vi "BWC_analogSamplePFFT.vi"() -> ()   [LabVIEW 2017]
uses:
  <vilib>/VirtualBench/_MSO Configure Analog Channel0.vi
  <vilib>/VirtualBench/_MSO Configure Timing8.vi
  <vilib>/measure/maspectr.llb/FFT Power Spectrum and PSD for N Chan.vi
  <vilib>/VirtualBench/VirtualBench.lvlib
  <vilib>/measure/NI_MAPro.lvlib
panel:
  in  "stop":bool
  in  "averaging parameters":T1={"averaging mode"=enum."No averaging", "weighting mode"=enum."Exponential", "number of averages"=10} {"number of averages" min=1}
  out "Power Spectrum / PSD":cluster{"f0":dbl, "df":dbl, "magnitude":dbl[]}[](graph)
  out "size(s)":i32
  in  "Auto Trigger":bool caption="Auto Trigger (False)"
  in  "Pretrigger Time (s)":dbl=0.5 caption="Pretrigger Time (s) (no change)"
  in  "Acquisition Time (s)":dbl=1.0 caption="Acquisition Time (s) (no change)"
  in  "Sample Rate":dbl=100000.0 caption="Sample Rate (no change)"
  in  "Vertical Range":dbl=1.0 caption="Vertical Range (no change)"
  in  "Vertical Offset":dbl caption="Vertical Offset (no change)"
  in  "Probe Attenuation":i32(ring)=1 caption="Probe Attenuation (no change)" items=["1x"=1, "10x"=10]
  in  "Vertical Coupling":i32(ring)=1 caption="Vertical Coupling (no change)" items=["AC", "DC"]
  in  "Enable Channel":bool=TRUE caption="Enable Channel (no change)"
  in  "Channel":tag
  out "Analog Waveforms":dynamicdata(graph)
  out "Error Out":errorcluster
  in  "Device Name":tag
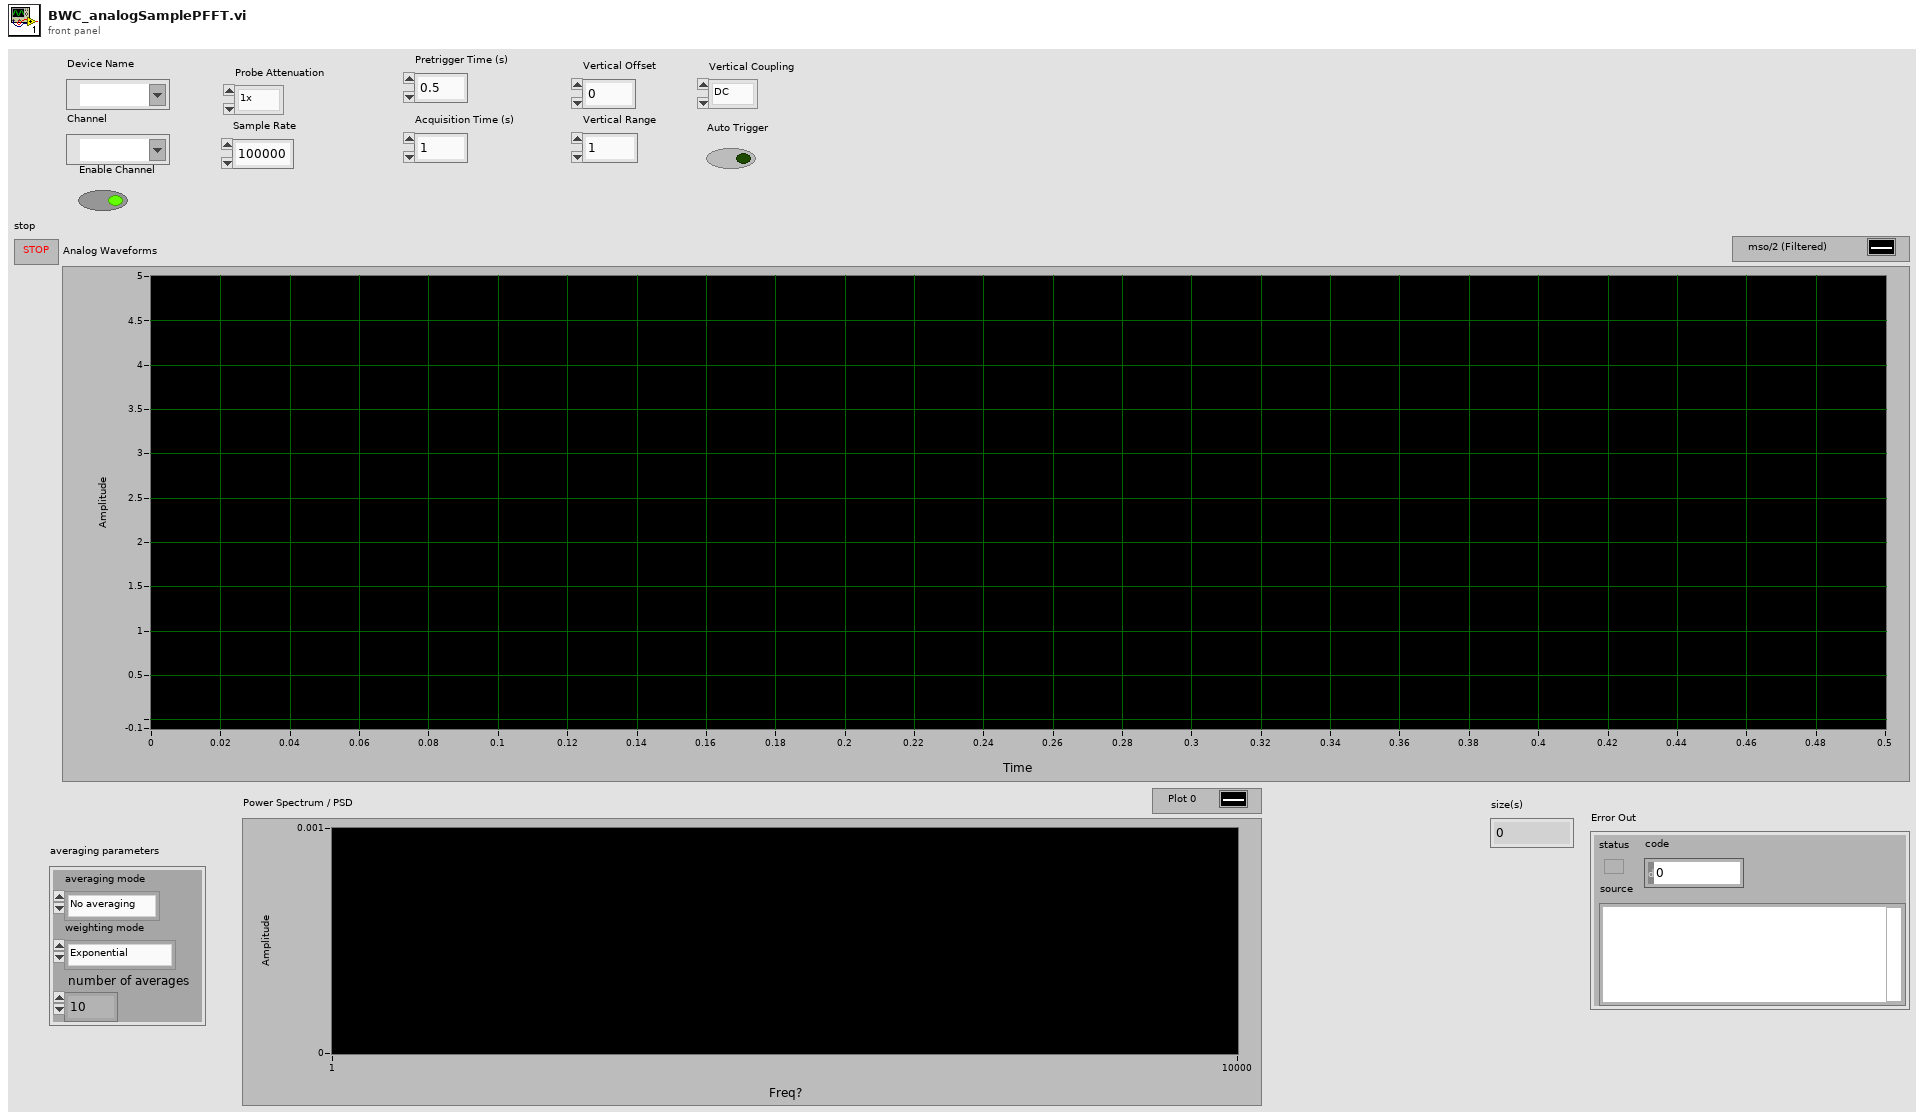
[diagram p1: front panel]
types:
  T1 = cluster{"averaging mode":enum16{"No averaging", "Vector averaging", "RMS averaging", "Peak hold"}, "weighting mode":enum16{"Linear", "Exponential"}, "number of averages":u32}
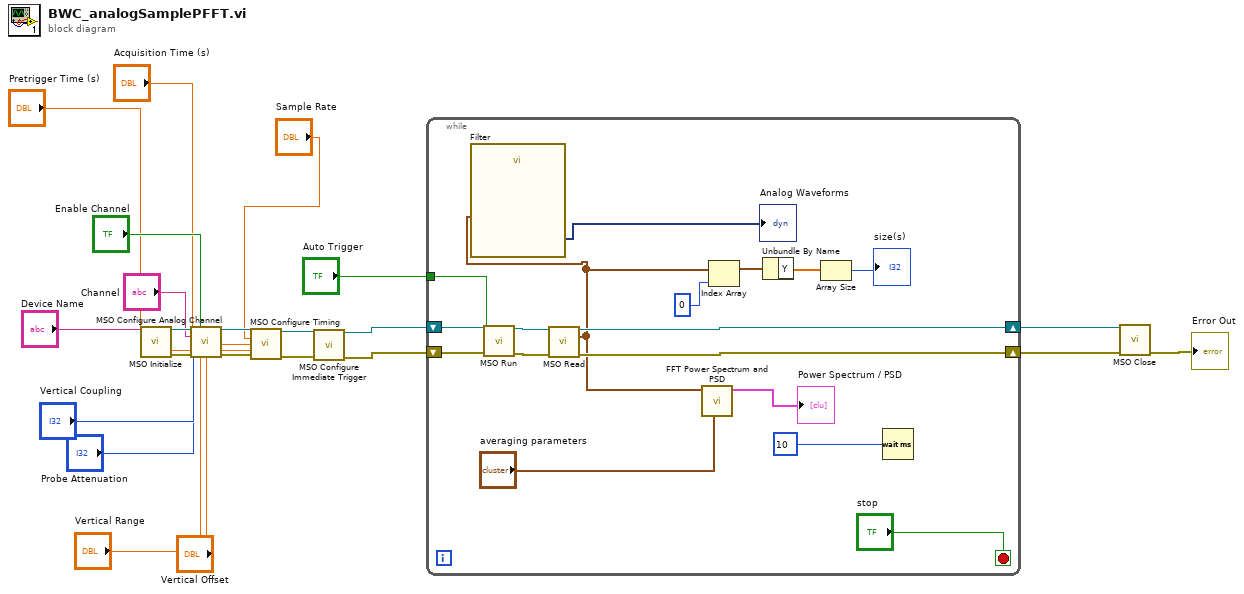
[diagram p0: block diagram]
diagram:
  n1 = call <vilib>:"MSO Initialize.vi"("Device Name"="Device Name") -> ("Instrument Handle Out"=w18:refnum<k21>, "Error Out"=w17:errorcluster)  [unwired: 13 in]
  n2 = call-poly <vilib>:"MSO Configure Analog Channel.vi"("Instrument Handle In"=w18, "Enable Channel"="Enable Channel", "Channel"="Channel", "Vertical Coupling"="Vertical Coupling", "Probe Attenuation"="Probe Attenuation", "Error In"=w17, "Vertical Range"="Vertical Range", "Vertical Offset"="Vertical Offset") -> ("Instrument Handle Out"=w15:refnum<k21>, "Error Out"=w12:errorcluster)  [unwired: 6 in]
  n3 = call-poly <vilib>:"MSO Configure Timing.vi"("Instrument Handle In"=w15, "Sample Rate"="Sample Rate", "Acquisition Time (s)"="Acquisition Time (s)", "Pretrigger Time (s)"="Pretrigger Time (s)", "Error In"=w12) -> ("Instrument Handle Out"=w14:refnum<k21>, "Error Out"=w11:errorcluster)  [unwired: 9 in]
  n4 = call <vilib>:"MSO Configure Immediate Trigger.vi"("Instrument Handle In"=w14, "Error In"=w11) -> ("Instrument Handle Out"=w13:refnum<k21>, "Error Out"=w10:errorcluster)  [unwired: 12 in]
  n5 = while {
    tunnel: "Auto Trigger" -> [w33]
    shift-right: [w39] -> w21
    shift-left: w13 -> [w37]
    shift-right: [w38] -> w20
    shift-left: w10 -> [w35]
    stop <- "stop" stop-if-true
    n6 = call <vilib>:"MSO Run.vi"("Instrument Handle In"=w37, "Auto Trigger"=w33, "Error In"=w35) -> ("Instrument Handle Out"=w36:refnum<k21>, "Error Out"=w34:errorcluster)  [unwired: 11 in]
    n7 = call <vilib>:"MSO Read.vi"("Instrument Handle In"=w36, "Error In"=w34) -> ("Instrument Handle Out"=w39:refnum<k21>, "Analog Waveforms"=w24:waveform(dbl)[], "Error Out"=w38:errorcluster)  [unwired: 8 in, 3 out]
    n8 = call "Filter"("Signal"=w24) -> ("Filtered Signal"=→"Analog Waveforms":dynamicdata)  [unwired: 9 in, 1 out]
    n9 = call-poly <vilib>:"FFT Power Spectrum and PSD.vi"("averaging parameters"="averaging parameters", "time signals"=w24) -> ("Power Spectrum / PSD"=→"Power Spectrum / PSD":cluster{"f0":dbl, "df":dbl, "magnitude":dbl[]}[])  [unwired: 6 in, 3 out]
    n10 = Index Array(array=w24, index=0) -> (element=w29:waveform(dbl))
    n11 = Unbundle By Name(w29) -> ("Y"=w28:dbl[])
    n12 = Array Size(array=w28) -> (size(s)=→"size(s)":i32)
    n13 = Wait (ms)(milliseconds to wait=u32 10) -> ()  [unwired: 1 out]
  }
  n14 = call <vilib>:"MSO Close.vi"("Instrument Handle In"=w21, "Error In"=w20) -> ("Error Out"=→"Error Out":errorcluster)  [unwired: 13 in]
